vi "RS_RTO1024_ConvIntoFormatString.vi"(6 "Mode":enum16{"Value", "Status"}(ring), 8 "Error In":errorcluster, 11 "input string":string) -> (0 "Error Out":errorcluster, 3 "output":string)   [LabVIEW 2018]
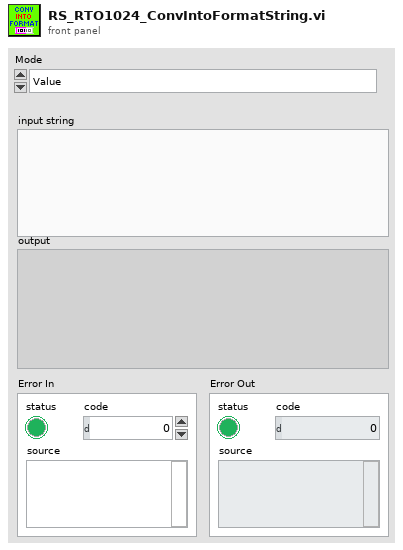
[diagram p1: front panel]
types:
  T1 = typedef "MLLC_Error.ctl" = errorcluster
  T2 = typedef "MLLC_Command.ctl" = string
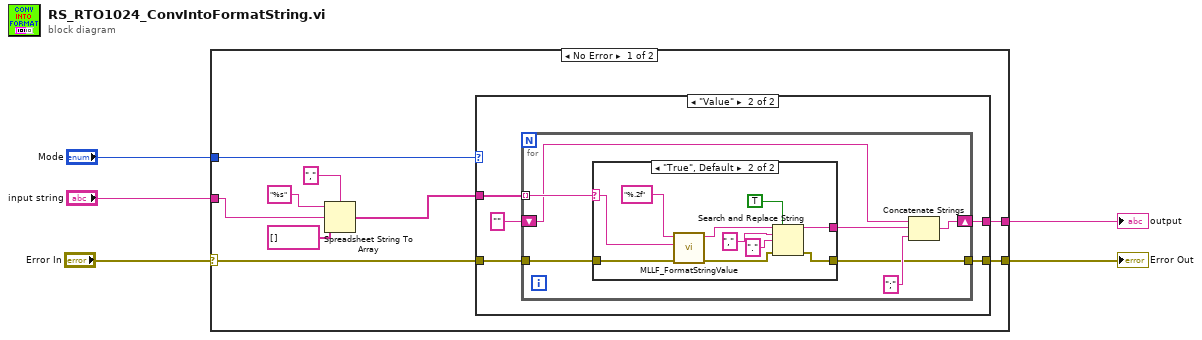
[diagram p0: block diagram]
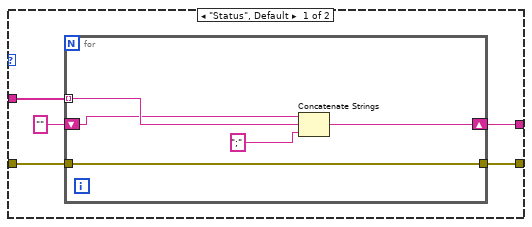
[diagram p2: hidden frame]
diagram:
  n1 = case shown="No Error" "Error In" {
    selector: "Error In" -> [w14 w49]
    tunnel: [w12 w49] -> w4
    tunnel: "input string" -> [w7 _]
    tunnel: [w13 _] -> w2
    tunnel: "Mode" -> [w11 _]
    frame No Error {
      n2 = Spreadsheet String To Array(delimiter (Tab)=",", format string="%s", spreadsheet string=w7, array type (2D Dbl)=string[] [] ("appended array")) -> (array=w6:string[])
      n3 = case shown="\"Value\"" w11 {
        tunnel: w14 -> [w16 w29]
        tunnel: [w18 w27] -> w13
        tunnel: [w17 w26] -> w12
        tunnel: w6 -> [w15 w25]
        frame "Status", Default {
          n4 = for {
            tunnel: w15 -> [w22] mode=indexing
            shift-right: [w24] -> w18
            shift-left: "" -> [w20]
            tunnel: w16 -> [w21]
            tunnel: [w21] -> w17
            n5 = Concatenate Strings(w20, w22, ";" ("string")) -> (w24:string)
          }
        }
        frame "Value" {
          n6 = for {
            tunnel: w25 -> [w31] mode=indexing
            shift-right: [w35] -> w27
            shift-left: "" -> [w30]
            tunnel: w29 -> [w36]
            tunnel: [w32] -> w26
            n7 = case shown="\"True\", Default" w31 {
              selector: w31 -> [w37 w39]
              tunnel: w36 -> [w38 w48]
              tunnel: [w37 w43] -> w33
              tunnel: [w38 w41] -> w32
              frame "NCAP" {
              }
              frame "True", Default {
                n8 = call "MLLF_FormatStringValue.vi"("error in"=w48, "String Value"=w39, "Format"="%.2f" ("format")) -> ("error out"=w42:T1, "String Value Formated"=w46:T2)  [unwired: 6 in, 1 out]
                n9 = Search and Replace String(replace all?=TRUE ("replace all? (F)"), input string=w46, search string=",", replace string="." ("replace string (\"\")"), error in=w42) -> (result string=w43:string, error out=w41:errorcluster)  [unwired: 3 in, 2 out]
              }
            }
            n10 = Concatenate Strings(w30, w33, ";" ("string")) -> (w35:string)
          }
        }
      }
    }
    frame Error {
    }
  }
  "Error Out" <- w4
  "output" <- w2
